vi "classeParCarton.vi"(11 "Tableau":string[][](array[string])=[["484147311015190508  ", "06.05.2015 09:48:00", "1866", "155915", "1", "1", "1", "11", "0"], ["484147311015190518  ", "06.05.2015 09:50:00", "1866", "155915", "1", "1", "1", "12", "0"], ["484147311015190505  ", "06.05.2015 09:38:00", "1866", "155915", "1", "1", "1", "5", "0"], ["484147311015190517  ", "06.05.2015 09:52:00", "1866", "155915", "1", "1", "1", "13", "0"], ["484147311015190506  ", "06.05.2015 09:50:00", "1866", "155915", "1", "1", "1", "12", "0"], ["484147311015190522  ", "06.05.2015 09:50:00", "1866", "155915", "1", "1", "1", "12", "0"], ["484147311015190533  ", "06.05.2015 09:41:00", "1866", "155915", "1", "1", "1", "7", "0"], ["484147311015190507  ", "06.05.2015 09:43:00", "1866", "155915", "1", "1", "1", "8", "0"], ["484147311015190550  ", "06.05.2015 09:50:00", "1866", "155915", "1", "1", "1", "12", "0"], ["484147311015190534  ", "06.05.2015 09:52:00", "1866", "155915", "1", "1", "1", "13", "0"], ["484147311015190535  ", "06.05.2015 09:40:00", "1866", "155915", "1", "1", "1", "6", "0"], ["484147311015190536  ", "06.05.2015 09:50:00", "1866", "155915", "1", "1", "1", "12", "0"], ["484147311015190537  ", "06.05.2015 09:53:00", "1866", "155915", "1", "1", "1", "13", "0"], ["484147311015190538  ", "06.05.2015 09:50:00", "1866", "155915", "1", "1", "1", "12", "0"], ["484147311015190551  ", "06.05.2015 09:53:00", "1866", "155915", "1", "1", "1", "13", "0"], ["484147311015190552  ", "06.05.2015 09:52:00", "1866", "155915", "1", "1", "1", "13", "0"], ["484147311015190539  ", "06.05.2015 09:53:00", "1866", "155915", "1", "1", "1", "13", "0"], ["484147311015190549  ", "06.05.2015 09:50:00", "1866", "155915", "1", "1", "1", "12", "0"], ["484147311015190540  ", "06.05.2015 09:38:00", "1866", "155915", "1", "1", "1", "5", "0"], ["484147311015190541  ", "06.05.2015 09:52:00", "1866", "155915", "1", "1", "1", "13", "0"], ["484147311015190527  ", "06.05.2015 09:50:00", "1866", "155915", "1", "1", "1", "12", "0"], ["484147311015190531  ", "06.05.2015 09:51:00", "1866", "155915", "1", "1", "1", "13", "0"], ["484147311015190525  ", "06.05.2015 09:41:00", "1866", "155915", "1", "1", "1", "7", "0"], ["484147311015190545  ", "06.05.2015 09:50:00", "1866", "155915", "1", "1", "1", "12", "0"], ["484147311015190546  ", "06.05.2015 09:53:00", "1866", "155915", "1", "1", "1", "13", "0"], ["484147311015190547  ", "06.05.2015 09:49:00", "1866", "155915", "1", "1", "1", "11", "0"], ["484147311015190521  ", "06.05.2015 09:48:00", "1866", "155915", "1", "1", "1", "11", "0"], ["484147311015190574  ", "06.05.2015 09:35:00", "1866", "155915", "1", "1", "1", "3", "0"], ["484147311015190548  ", "06.05.2015 09:38:00", "1866", "155915", "1", "1", "1", "5", "0"], ["484147311015190520  ", "06.05.2015 09:34:00", "1866", "155915", "1", "1", "1", "2", "0"], ["484147311015190577  ", "06.05.2015 09:32:00", "1866", "155915", "1", "1", "1", "1", "0"], ["484147311015190573  ", "06.05.2015 09:37:00", "1866", "155915", "1", "1", "1", "4", "0"], ["484147311015190572  ", "06.05.2015 09:31:00", "1866", "155915", "1", "1", "1", "1", "0"], ["484147311015190569  ", "06.05.2015 09:39:00", "1866", "155915", "1", "1", "1", "6", "0"], ["484147311015190501  ", "06.05.2015 09:40:00", "1866", "155915", "1", "1", "1", "6", "0"], ["484147311015190503  ", "06.05.2015 09:39:00", "1866", "155915", "1", "1", "1", "6", "0"], ["484147311015190584  ", "06.05.2015 09:38:00", "1866", "155915", "1", "1", "1", "5", "0"], ["484147311015190583  ", "06.05.2015 09:32:00", "1866", "155915", "1", "1", "1", "1", "0"], ["484147311015190568  ", "06.05.2015 09:50:00", "1866", "155915", "1", "1", "1", "12", "0"], ["484147311015190567  ", "06.05.2015 09:40:00", "1866", "155915", "1", "1", "1", "6", "0"], ["484147311015190519  ", "06.05.2015 09:34:00", "1866", "155915", "1", "1", "1", "2", "0"], ["484147311015190566  ", "06.05.2015 09:48:00", "1866", "155915", "1", "1", "1", "11", "0"], ["484147311015190565  ", "06.05.2015 09:34:00", "1866", "155915", "1", "1", "1", "2", "0"], ["484147311015190581  ", "06.05.2015 09:46:00", "1866", "155915", "1", "1", "1", "10", "0"], ["484147311015190564  ", "06.05.2015 09:32:00", "1866", "155915", "1", "1", "1", "1", "0"], ["484147311015190575  ", "06.05.2015 09:42:00", "1866", "155915", "1", "1", "1", "7", "0"], ["484147311015190576  ", "06.05.2015 09:34:00", "1866", "155915", "1", "1", "1", "2", "0"], ["484147311015190578  ", "06.05.2015 09:34:00", "1866", "155915", "1", "1", "1", "2", "0"], ["484147311015190563  ", "06.05.2015 09:43:00", "1866", "155915", "1", "1", "1", "8", "0"], ["484147311015190561  ", "06.05.2015 09:45:00", "1866", "155915", "1", "1", "1", "9", "0"], ["484147311015190579  ", "06.05.2015 09:32:00", "1866", "155915", "1", "1", "1", "1", "0"], ["484147311015190562  ", "06.05.2015 09:32:00", "1866", "155915", "1", "1", "1", "1", "0"], ["484147311015190582  ", "06.05.2015 09:42:00", "1866", "155915", "1", "1", "1", "8", "0"], ["484147311015190560  ", "06.05.2015 09:32:00", "1866", "155915", "1", "1", "1", "1", "0"], ["484147311015190587  ", "06.05.2015 09:34:00", "1866", "155915", "1", "1", "1", "2", "0"], ["484147311015190590  ", "06.05.2015 09:34:00", "1866", "155915", "1", "1", "1", "2", "0"], ["484147311015190589  ", "06.05.2015 09:43:00", "1866", "155915", "1", "1", "1", "8", "0"], ["484147311015190559  ", "06.05.2015 09:33:00", "1866", "155915", "1", "1", "1", "1", "0"], ["484147311015190585  ", "06.05.2015 09:33:00", "1866", "155915", "1", "1", "1", "2", "0"], ["484147311015190558  ", "06.05.2015 09:42:00", "1866", "155915", "1", "1", "1", "7", "0"], ["484147311015190586  ", "06.05.2015 09:43:00", "1866", "155915", "1", "1", "1", "8", "0"], ["484147311015190588  ", "06.05.2015 09:45:00", "1866", "155915", "1", "1", "1", "9", "0"], ["484147311015190603  ", "06.05.2015 09:38:00", "1866", "155915", "1", "1", "1", "5", "0"], ["484147311015190594  ", "06.05.2015 09:33:00", "1866", "155915", "1", "1", "1", "2", "0"], ["484147311015190593  ", "06.05.2015 09:33:00", "1866", "155915", "1", "1", "1", "2", "0"], ["484147311015190604  ", "06.05.2015 09:39:00", "1866", "155915", "1", "1", "1", "6", "0"], ["484147311015190595  ", "06.05.2015 09:34:00", "1866", "155915", "1", "1", "1", "2", "0"], ["484147311015190596  ", "06.05.2015 09:32:00", "1866", "155915", "1", "1", "1", "1", "0"], ["484147311015190597  ", "06.05.2015 09:32:00", "1866", "155915", "1", "1", "1", "1", "0"], ["484147311015190606  ", "06.05.2015 09:31:00", "1866", "155915", "1", "1", "1", "1", "0"], ["484147311015190598  ", "06.05.2015 09:32:00", "1866", "155915", "1", "1", "1", "1", "0"], ["484147311015190605  ", "06.05.2015 09:35:00", "1866", "155915", "1", "1", "1", "3", "0"], ["484147311015190599  ", "06.05.2015 09:32:00", "1866", "155915", "1", "1", "1", "1", "0"], ["484147311015190608  ", "06.05.2015 09:34:00", "1866", "155915", "1", "1", "1", "2", "0"], ["484147311015190600  ", "06.05.2015 09:32:00", "1866", "155915", "1", "1", "1", "1", "0"], ["484147311015190556  ", "06.05.2015 09:31:00", "1866", "155915", "1", "1", "1", "1", "0"], ["484147311015190555  ", "06.05.2015 09:32:00", "1866", "155915", "1", "1", "1", "1", "0"], ["484147311015190602  ", "06.05.2015 09:34:00", "1866", "155915", "1", "1", "1", "2", "0"], ["484147311015190609  ", "06.05.2015 09:33:00", "1866", "155915", "1", "1", "1", "2", "0"], ["484147311015190610  ", "06.05.2015 09:32:00", "1866", "155915", "1", "1", "1", "1", "0"], ["484147311015190611  ", "06.05.2015 09:33:00", "1866", "155915", "1", "1", "1", "2", "0"], ["484147311015190554  ", "06.05.2015 09:38:00", "1866", "155915", "1", "1", "1", "5", "0"], ["484147311015190613  ", "06.05.2015 09:40:00", "1866", "155915", "1", "1", "1", "6", "0"], ["484147311015190612  ", "06.05.2015 09:55:00", "1866", "155915", "1", "1", "1", "14", "0"], ["484147311015190623  ", "06.05.2015 09:32:00", "1866", "155915", "1", "1", "1", "1", "0"], ["484147311015190614  ", "06.05.2015 09:41:00", "1866", "155915", "1", "1", "1", "7", "0"], ["484147311015190625  ", "06.05.2015 09:32:00", "1866", "155915", "1", "1", "1", "1", "0"], ["484147311015190615  ", "06.05.2015 09:35:00", "1866", "155915", "1", "1", "1", "3", "0"], ["484147311015190617  ", "06.05.2015 09:37:00", "1866", "155915", "1", "1", "1", "4", "0"], ["484147311015190616  ", "06.05.2015 09:41:00", "1866", "155915", "1", "1", "1", "7", "0"], ["484147311015190618  ", "06.05.2015 09:37:00", "1866", "155915", "1", "1", "1", "4", "0"], ["484147311015190619  ", "06.05.2015 09:39:00", "1866", "155915", "1", "1", "1", "6", "0"], ["484147311015190627  ", "06.05.2015 09:40:00", "1866", "155915", "1", "1", "1", "6", "0"], ["484147311015190620  ", "06.05.2015 09:46:00", "1866", "155915", "1", "1", "1", "10", "0"], ["484147311015190629  ", "06.05.2015 09:46:00", "1866", "155915", "1", "1", "1", "10", "0"], ["484147311015190633  ", "06.05.2015 09:38:00", "1866", "155915", "1", "1", "1", "5", "0"], ["484147311015190601  ", "06.05.2015 09:46:00", "1866", "155915", "1", "1", "1", "10", "0"], ["484147311015190635  ", "06.05.2015 09:39:00", "1866", "155915", "1", "1", "1", "6", "0"], ["484147311015190637  ", "06.05.2015 09:45:00", "1866", "155915", "1", "1", "1", "9", "0"], ["484147311015190636  ", "06.05.2015 09:49:00", "1866", "155915", "1", "1", "1", "11", "0"], ["484147311015190667  ", "06.05.2015 09:39:00", "1866", "155915", "1", "1", "1", "6", "0"], ["484147311015180237  ", "06.05.2015 10:00:00", "1866", "155915", "1", "1", "1", "16", "0"], ["484147311015180267  ", "06.05.2015 09:58:00", "1866", "155915", "1", "1", "1", "15", "0"], ["484147311015180419  ", "06.05.2015 10:01:00", "1866", "155915", "1", "1", "1", "16", "0"], ["484147311015180644  ", "06.05.2015 09:50:00", "1866", "155915", "1", "1", "1", "12", "0"], ["484147311015180688  ", "06.05.2015 10:01:00", "1866", "155915", "1", "1", "1", "16", "0"], ["484147311015180709  ", "06.05.2015 10:01:00", "1866", "155915", "1", "1", "1", "16", "0"], ["484147311015180701  ", "06.05.2015 09:55:00", "1866", "155915", "1", "1", "1", "14", "0"], ["484147311015180703  ", "06.05.2015 10:01:00", "1866", "155915", "1", "1", "1", "16", "0"], ["484147311015180707  ", "06.05.2015 09:56:00", "1866", "155915", "1", "1", "1", "14", "0"], ["484147311015180718  ", "06.05.2015 10:00:00", "1866", "155915", "1", "1", "1", "16", "0"], ["484147311015180717  ", "06.05.2015 09:57:00", "1866", "155915", "1", "1", "1", "15", "0"], ["484147311015180715  ", "06.05.2015 09:55:00", "1866", "155915", "1", "1", "1", "14", "0"], ["484147311015180726  ", "06.05.2015 09:56:00", "1866", "155915", "1", "1", "1", "14", "0"], ["484147311015180728  ", "06.05.2015 09:56:00", "1866", "155915", "1", "1", "1", "14", "0"], ["484147311015180737  ", "06.05.2015 10:00:00", "1866", "155915", "1", "1", "1", "16", "0"], ["484147311015190019  ", "06.05.2015 09:33:00", "1866", "155915", "1", "1", "1", "2", "0"], ["484147311015190016  ", "06.05.2015 09:47:00", "1866", "155915", "1", "1", "1", "10", "0"], ["484147311015190022  ", "06.05.2015 09:43:00", "1866", "155915", "1", "1", "1", "8", "0"], ["484147311015190027  ", "06.05.2015 09:48:00", "1866", "155915", "1", "1", "1", "11", "0"], ["484147311015190035  ", "06.05.2015 10:00:00", "1866", "155915", "1", "1", "1", "16", "0"], ["484147311015190044  ", "06.05.2015 10:01:00", "1866", "155915", "1", "1", "1", "16", "0"], ["484147311015190046  ", "06.05.2015 09:58:00", "1866", "155915", "1", "1", "1", "15", "0"], ["484147311015190045  ", "06.05.2015 09:57:00", "1866", "155915", "1", "1", "1", "15", "0"], ["484147311015190057  ", "06.05.2015 09:58:00", "1866", "155915", "1", "1", "1", "15", "0"], ["484147311015190055  ", "06.05.2015 09:33:00", "1866", "155915", "1", "1", "1", "2", "0"], ["484147311015190056  ", "06.05.2015 09:58:00", "1866", "155915", "1", "1", "1", "15", "0"], ["484147311015190052  ", "06.05.2015 09:56:00", "1866", "155915", "1", "1", "1", "14", "0"], ["484147311015190059  ", "06.05.2015 09:58:00", "1866", "155915", "1", "1", "1", "15", "0"], ["484147311015190060  ", "06.05.2015 09:59:00", "1866", "155915", "1", "1", "1", "15", "0"], ["484147311015190064  ", "06.05.2015 09:58:00", "1866", "155915", "1", "1", "1", "15", "0"], ["484147311015190068  ", "06.05.2015 09:47:00", "1866", "155915", "1", "1", "1", "10", "0"], ["484147311015190084  ", "06.05.2015 09:59:00", "1866", "155915", "1", "1", "1", "15", "0"], ["484147311015190081  ", "06.05.2015 09:59:00", "1866", "155915", "1", "1", "1", "15", "0"], ["484147311015190082  ", "06.05.2015 10:00:00", "1866", "155915", "1", "1", "1", "16", "0"], ["484147311015190098  ", "06.05.2015 09:56:00", "1866", "155915", "1", "1", "1", "14", "0"], ["484147311015190096  ", "06.05.2015 09:59:00", "1866", "155915", "1", "1", "1", "15", "0"], ["484147311015190091  ", "06.05.2015 09:56:00", "1866", "155915", "1", "1", "1", "14", "0"], ["484147311015190118  ", "06.05.2015 09:55:00", "1866", "155915", "1", "1", "1", "14", "0"], ["484147311015190117  ", "06.05.2015 09:40:00", "1866", "155915", "1", "1", "1", "6", "0"], ["484147311015190113  ", "06.05.2015 10:00:00", "1866", "155915", "1", "1", "1", "16", "0"], ["484147311015190111  ", "06.05.2015 10:01:00", "1866", "155915", "1", "1", "1", "16", "0"], ["484147311015190108  ", "06.05.2015 10:00:00", "1866", "155915", "1", "1", "1", "16", "0"], ["484147311015190135  ", "06.05.2015 09:59:00", "1866", "155915", "1", "1", "1", "15", "0"], ["484147311015190133  ", "06.05.2015 10:00:00", "1866", "155915", "1", "1", "1", "16", "0"], ["484147311015190131  ", "06.05.2015 09:41:00", "1866", "155915", "1", "1", "1", "7", "0"], ["484147311015190129  ", "06.05.2015 09:56:00", "1866", "155915", "1", "1", "1", "14", "0"], ["484147311015190123  ", "06.05.2015 09:57:00", "1866", "155915", "1", "1", "1", "15", "0"], ["484147311015190121  ", "06.05.2015 09:57:00", "1866", "155915", "1", "1", "1", "15", "0"], ["484147311015190124  ", "06.05.2015 09:58:00", "1866", "155915", "1", "1", "1", "15", "0"], ["484147311015190126  ", "06.05.2015 10:01:00", "1866", "155915", "1", "1", "1", "16", "0"], ["484147311015190132  ", "06.05.2015 10:00:00", "1866", "155915", "1", "1", "1", "16", "0"], ["484147311015190150  ", "06.05.2015 09:59:00", "1866", "155915", "1", "1", "1", "15", "0"], ["484147311015190146  ", "06.05.2015 09:58:00", "1866", "155915", "1", "1", "1", "15", "0"], ["484147311015190149  ", "06.05.2015 09:57:00", "1866", "155915", "1", "1", "1", "15", "0"], ["484147311015190145  ", "06.05.2015 09:48:00", "1866", "155915", "1", "1", "1", "11", "0"], ["484147311015190159  ", "06.05.2015 09:57:00", "1866", "155915", "1", "1", "1", "15", "0"], ["484147311015190183  ", "06.05.2015 09:56:00", "1866", "155915", "1", "1", "1", "14", "0"], ["484147311015190181  ", "06.05.2015 09:56:00", "1866", "155915", "1", "1", "1", "14", "0"], ["484147311015190180  ", "06.05.2015 09:55:00", "1866", "155915", "1", "1", "1", "14", "0"], ["484147311015190179  ", "06.05.2015 10:01:00", "1866", "155915", "1", "1", "1", "16", "0"], ["484147311015190177  ", "06.05.2015 09:48:00", "1866", "155915", "1", "1", "1", "11", "0"], ["484147311015190168  ", "06.05.2015 09:58:00", "1866", "155915", "1", "1", "1", "15", "0"], ["484147311015190173  ", "06.05.2015 09:56:00", "1866", "155915", "1", "1", "1", "14", "0"], ["484147311015190175  ", "06.05.2015 09:58:00", "1866", "155915", "1", "1", "1", "15", "0"], ["484147311015190193  ", "06.05.2015 10:01:00", "1866", "155915", "1", "1", "1", "16", "0"], ["484147311015190194  ", "06.05.2015 09:58:00", "1866", "155915", "1", "1", "1", "15", "0"], ["484147311015190197  ", "06.05.2015 10:01:00", "1866", "155915", "1", "1", "1", "16", "0"], ["484147311015190196  ", "06.05.2015 09:59:00", "1866", "155915", "1", "1", "1", "15", "0"], ["484147311015190198  ", "06.05.2015 09:56:00", "1866", "155915", "1", "1", "1", "14", "0"], ["484147311015190188  ", "06.05.2015 09:59:00", "1866", "155915", "1", "1", "1", "15", "0"], ["484147311015190218  ", "06.05.2015 09:39:00", "1866", "155915", "1", "1", "1", "5", "0"], ["484147311015190215  ", "06.05.2015 10:01:00", "1866", "155915", "1", "1", "1", "16", "0"], ["484147311015190290  ", "06.05.2015 09:42:00", "1866", "155915", "1", "1", "1", "7", "0"], ["484147311015190288  ", "06.05.2015 09:50:00", "1866", "155915", "1", "1", "1", "12", "0"], ["484147311015190297  ", "06.05.2015 09:46:00", "1866", "155915", "1", "1", "1", "10", "0"], ["484147311015190314  ", "06.05.2015 09:45:00", "1866", "155915", "1", "1", "1", "9", "0"], ["484147311015190313  ", "06.05.2015 09:42:00", "1866", "155915", "1", "1", "1", "8", "0"], ["484147311015190312  ", "06.05.2015 09:41:00", "1866", "155915", "1", "1", "1", "7", "0"], ["484147311015190311  ", "06.05.2015 09:45:00", "1866", "155915", "1", "1", "1", "9", "0"], ["484147311015190310  ", "06.05.2015 09:42:00", "1866", "155915", "1", "1", "1", "7", "0"], ["484147311015190303  ", "06.05.2015 09:42:00", "1866", "155915", "1", "1", "1", "7", "0"], ["484147311015190306  ", "06.05.2015 09:42:00", "1866", "155915", "1", "1", "1", "8", "0"], ["484147311015190305  ", "06.05.2015 09:45:00", "1866", "155915", "1", "1", "1", "9", "0"], ["484147311015190304  ", "06.05.2015 09:45:00", "1866", "155915", "1", "1", "1", "9", "0"], ["484147311015190307  ", "06.05.2015 09:42:00", "1866", "155915", "1", "1", "1", "8", "0"], ["484147311015190308  ", "06.05.2015 09:41:00", "1866", "155915", "1", "1", "1", "7", "0"], ["484147311015190309  ", "06.05.2015 09:45:00", "1866", "155915", "1", "1", "1", "9", "0"], ["484147311015190326  ", "06.05.2015 09:42:00", "1866", "155915", "1", "1", "1", "7", "0"], ["484147311015190328  ", "06.05.2015 09:34:00", "1866", "155915", "1", "1", "1", "2", "0"], ["484147311015190329  ", "06.05.2015 09:40:00", "1866", "155915", "1", "1", "1", "6", "0"], ["484147311015190330  ", "06.05.2015 09:46:00", "1866", "155915", "1", "1", "1", "10", "0"], ["484147311015190331  ", "06.05.2015 09:45:00", "1866", "155915", "1", "1", "1", "9", "0"], ["484147311015190317  ", "06.05.2015 09:43:00", "1866", "155915", "1", "1", "1", "8", "0"], ["484147311015190316  ", "06.05.2015 09:45:00", "1866", "155915", "1", "1", "1", "9", "0"], ["484147311015190318  ", "06.05.2015 09:49:00", "1866", "155915", "1", "1", "1", "12", "0"], ["484147311015190320  ", "06.05.2015 09:34:00", "1866", "155915", "1", "1", "1", "2", "0"], ["484147311015190321  ", "06.05.2015 09:46:00", "1866", "155915", "1", "1", "1", "10", "0"], ["484147311015190322  ", "06.05.2015 09:45:00", "1866", "155915", "1", "1", "1", "9", "0"], ["484147311015190323  ", "06.05.2015 09:45:00", "1866", "155915", "1", "1", "1", "9", "0"], ["484147311015190347  ", "06.05.2015 09:43:00", "1866", "155915", "1", "1", "1", "8", "0"], ["484147311015190346  ", "06.05.2015 09:46:00", "1866", "155915", "1", "1", "1", "10", "0"], ["484147311015190345  ", "06.05.2015 09:36:00", "1866", "155915", "1", "1", "1", "3", "0"], ["484147311015190344  ", "06.05.2015 09:45:00", "1866", "155915", "1", "1", "1", "9", "0"], ["484147311015190343  ", "06.05.2015 09:44:00", "1866", "155915", "1", "1", "1", "9", "0"], ["484147311015190341  ", "06.05.2015 09:44:00", "1866", "155915", "1", "1", "1", "9", "0"], ["484147311015190340  ", "06.05.2015 09:46:00", "1866", "155915", "1", "1", "1", "10", "0"], ["484147311015190332  ", "06.05.2015 09:45:00", "1866", "155915", "1", "1", "1", "9", "0"], ["484147311015190333  ", "06.05.2015 09:35:00", "1866", "155915", "1", "1", "1", "3", "0"], ["484147311015190334  ", "06.05.2015 09:45:00", "1866", "155915", "1", "1", "1", "9", "0"], ["484147311015190335  ", "06.05.2015 09:46:00", "1866", "155915", "1", "1", "1", "10", "0"], ["484147311015190336  ", "06.05.2015 09:45:00", "1866", "155915", "1", "1", "1", "9", "0"], ["484147311015190337  ", "06.05.2015 09:33:00", "1866", "155915", "1", "1", "1", "2", "0"], ["484147311015190339  ", "06.05.2015 09:42:00", "1866", "155915", "1", "1", "1", "7", "0"], ["484147311015190348  ", "06.05.2015 09:43:00", "1866", "155915", "1", "1", "1", "8", "0"], ["484147311015190349  ", "06.05.2015 09:46:00", "1866", "155915", "1", "1", "1", "10", "0"], ["484147311015190350  ", "06.05.2015 09:43:00", "1866", "155915", "1", "1", "1", "8", "0"], ["484147311015190351  ", "06.05.2015 09:45:00", "1866", "155915", "1", "1", "1", "9", "0"], ["484147311015190352  ", "06.05.2015 09:45:00", "1866", "155915", "1", "1", "1", "9", "0"], ["484147311015190353  ", "06.05.2015 09:33:00", "1866", "155915", "1", "1", "1", "2", "0"], ["484147311015190354  ", "06.05.2015 09:35:00", "1866", "155915", "1", "1", "1", "3", "0"], ["484147311015190360  ", "06.05.2015 09:37:00", "1866", "155915", "1", "1", "1", "4", "0"], ["484147311015190355  ", "06.05.2015 09:32:00", "1866", "155915", "1", "1", "1", "1", "0"], ["484147311015190361  ", "06.05.2015 09:37:00", "1866", "155915", "1", "1", "1", "4", "0"], ["484147311015190356  ", "06.05.2015 09:41:00", "1866", "155915", "1", "1", "1", "7", "0"], ["484147311015190362  ", "06.05.2015 09:39:00", "1866", "155915", "1", "1", "1", "5", "0"], ["484147311015190357  ", "06.05.2015 09:37:00", "1866", "155915", "1", "1", "1", "4", "0"], ["484147311015190363  ", "06.05.2015 09:36:00", "1866", "155915", "1", "1", "1", "4", "0"], ["484147311015190358  ", "06.05.2015 09:44:00", "1866", "155915", "1", "1", "1", "9", "0"], ["484147311015190372  ", "06.05.2015 09:35:00", "1866", "155915", "1", "1", "1", "3", "0"], ["484147311015190371  ", "06.05.2015 09:36:00", "1866", "155915", "1", "1", "1", "4", "0"], ["484147311015190373  ", "06.05.2015 09:36:00", "1866", "155915", "1", "1", "1", "3", "0"], ["484147311015190370  ", "06.05.2015 09:41:00", "1866", "155915", "1", "1", "1", "7", "0"], ["484147311015190381  ", "06.05.2015 09:37:00", "1866", "155915", "1", "1", "1", "4", "0"], ["484147311015190380  ", "06.05.2015 09:36:00", "1866", "155915", "1", "1", "1", "3", "0"], ["484147311015190386  ", "06.05.2015 09:35:00", "1866", "155915", "1", "1", "1", "3", "0"], ["484147311015190382  ", "06.05.2015 09:45:00", "1866", "155915", "1", "1", "1", "9", "0"], ["484147311015190387  ", "06.05.2015 09:35:00", "1866", "155915", "1", "1", "1", "3", "0"], ["484147311015190369  ", "06.05.2015 09:41:00", "1866", "155915", "1", "1", "1", "7", "0"], ["484147311015190375  ", "06.05.2015 09:48:00", "1866", "155915", "1", "1", "1", "11", "0"], ["484147311015190376  ", "06.05.2015 09:36:00", "1866", "155915", "1", "1", "1", "3", "0"], ["484147311015190367  ", "06.05.2015 09:40:00", "1866", "155915", "1", "1", "1", "6", "0"], ["484147311015190377  ", "06.05.2015 09:40:00", "1866", "155915", "1", "1", "1", "6", "0"], ["484147311015190399  ", "06.05.2015 09:48:00", "1866", "155915", "1", "1", "1", "11", "0"], ["484147311015190395  ", "06.05.2015 09:49:00", "1866", "155915", "1", "1", "1", "12", "0"], ["484147311015190397  ", "06.05.2015 09:35:00", "1866", "155915", "1", "1", "1", "3", "0"], ["484147311015190378  ", "06.05.2015 09:39:00", "1866", "155915", "1", "1", "1", "6", "0"], ["484147311015190364  ", "06.05.2015 09:39:00", "1866", "155915", "1", "1", "1", "5", "0"], ["484147311015190393  ", "06.05.2015 09:40:00", "1866", "155915", "1", "1", "1", "6", "0"], ["484147311015190379  ", "06.05.2015 09:40:00", "1866", "155915", "1", "1", "1", "6", "0"], ["484147311015190389  ", "06.05.2015 09:40:00", "1866", "155915", "1", "1", "1", "6", "0"], ["484147311015190365  ", "06.05.2015 09:39:00", "1866", "155915", "1", "1", "1", "5", "0"], ["484147311015190412  ", "06.05.2015 09:38:00", "1866", "155915", "1", "1", "1", "5", "0"], ["484147311015190411  ", "06.05.2015 09:40:00", "1866", "155915", "1", "1", "1", "6", "0"], ["484147311015190409  ", "06.05.2015 09:38:00", "1866", "155915", "1", "1", "1", "5", "0"], ["484147311015190408  ", "06.05.2015 09:41:00", "1866", "155915", "1", "1", "1", "7", "0"], ["484147311015190407  ", "06.05.2015 09:55:00", "1866", "155915", "1", "1", "1", "14", "0"], ["484147311015190391  ", "06.05.2015 09:53:00", "1866", "155915", "1", "1", "1", "13", "0"], ["484147311015190400  ", "06.05.2015 09:35:00", "1866", "155915", "1", "1", "1", "3", "0"], ["484147311015190406  ", "06.05.2015 09:48:00", "1866", "155915", "1", "1", "1", "11", "0"], ["484147311015190426  ", "06.05.2015 09:49:00", "1866", "155915", "1", "1", "1", "12", "0"], ["484147311015190425  ", "06.05.2015 09:38:00", "1866", "155915", "1", "1", "1", "5", "0"], ["484147311015190427  ", "06.05.2015 09:42:00", "1866", "155915", "1", "1", "1", "7", "0"], ["484147311015190405  ", "06.05.2015 09:47:00", "1866", "155915", "1", "1", "1", "10", "0"], ["484147311015190430  ", "06.05.2015 09:35:00", "1866", "155915", "1", "1", "1", "3", "0"], ["484147311015190429  ", "06.05.2015 09:53:00", "1866", "155915", "1", "1", "1", "13", "0"], ["484147311015190410  ", "06.05.2015 09:47:00", "1866", "155915", "1", "1", "1", "10", "0"], ["484147311015190401  ", "06.05.2015 09:48:00", "1866", "155915", "1", "1", "1", "11", "0"], ["484147311015190404  ", "06.05.2015 09:37:00", "1866", "155915", "1", "1", "1", "4", "0"], ["484147311015190396  ", "06.05.2015 09:55:00", "1866", "155915", "1", "1", "1", "14", "0"], ["484147311015190394  ", "06.05.2015 09:38:00", "1866", "155915", "1", "1", "1", "5", "0"], ["484147311015190402  ", "06.05.2015 09:38:00", "1866", "155915", "1", "1", "1", "5", "0"], ["484147311015190390  ", "06.05.2015 09:37:00", "1866", "155915", "1", "1", "1", "4", "0"], ["484147311015190388  ", "06.05.2015 09:39:00", "1866", "155915", "1", "1", "1", "5", "0"], ["484147311015190436  ", "06.05.2015 09:42:00", "1866", "155915", "1", "1", "1", "8", "0"], ["484147311015190433  ", "06.05.2015 09:55:00", "1866", "155915", "1", "1", "1", "14", "0"], ["484147311015190434  ", "06.05.2015 09:41:00", "1866", "155915", "1", "1", "1", "7", "0"], ["484147311015190438  ", "06.05.2015 09:53:00", "1866", "155915", "1", "1", "1", "13", "0"], ["484147311015190392  ", "06.05.2015 09:55:00", "1866", "155915", "1", "1", "1", "14", "0"], ["484147311015190432  ", "06.05.2015 09:41:00", "1866", "155915", "1", "1", "1", "7", "0"], ["484147311015190431  ", "06.05.2015 09:55:00", "1866", "155915", "1", "1", "1", "14", "0"], ["484147311015190435  ", "06.05.2015 09:38:00", "1866", "155915", "1", "1", "1", "5", "0"], ["484147311015190422  ", "06.05.2015 09:54:00", "1866", "155915", "1", "1", "1", "14", "0"], ["484147311015190423  ", "06.05.2015 09:55:00", "1866", "155915", "1", "1", "1", "14", "0"], ["484147311015190421  ", "06.05.2015 09:41:00", "1866", "155915", "1", "1", "1", "7", "0"], ["484147311015190420  ", "06.05.2015 09:37:00", "1866", "155915", "1", "1", "1", "4", "0"], ["484147311015190424  ", "06.05.2015 09:52:00", "1866", "155915", "1", "1", "1", "13", "0"], ["484147311015190418  ", "06.05.2015 09:52:00", "1866", "155915", "1", "1", "1", "13", "0"], ["484147311015190419  ", "06.05.2015 09:38:00", "1866", "155915", "1", "1", "1", "5", "0"], ["484147311015190417  ", "06.05.2015 09:46:00", "1866", "155915", "1", "1", "1", "10", "0"], ["484147311015190439  ", "06.05.2015 09:53:00", "1866", "155915", "1", "1", "1", "13", "0"], ["484147311015190416  ", "06.05.2015 09:35:00", "1866", "155915", "1", "1", "1", "3", "0"], ["484147311015190414  ", "06.05.2015 09:49:00", "1866", "155915", "1", "1", "1", "11", "0"], ["484147311015190441  ", "06.05.2015 09:40:00", "1866", "155915", "1", "1", "1", "6", "0"], ["484147311015190415  ", "06.05.2015 09:52:00", "1866", "155915", "1", "1", "1", "13", "0"], ["484147311015190442  ", "06.05.2015 09:52:00", "1866", "155915", "1", "1", "1", "13", "0"], ["484147311015190440  ", "06.05.2015 09:36:00", "1866", "155915", "1", "1", "1", "4", "0"], ["484147311015190443  ", "06.05.2015 09:54:00", "1866", "155915", "1", "1", "1", "14", "0"], ["484147311015190413  ", "06.05.2015 09:37:00", "1866", "155915", "1", "1", "1", "4", "0"], ["484147311015190446  ", "06.05.2015 09:37:00", "1866", "155915", "1", "1", "1", "4", "0"], ["484147311015190444  ", "06.05.2015 09:53:00", "1866", "155915", "1", "1", "1", "13", "0"], ["484147311015190466  ", "06.05.2015 09:43:00", "1866", "155915", "1", "1", "1", "8", "0"], ["484147311015190437  ", "06.05.2015 09:40:00", "1866", "155915", "1", "1", "1", "6", "0"], ["484147311015190463  ", "06.05.2015 09:42:00", "1866", "155915", "1", "1", "1", "7", "0"], ["484147311015190459  ", "06.05.2015 09:48:00", "1866", "155915", "1", "1", "1", "11", "0"], ["484147311015190462  ", "06.05.2015 09:53:00", "1866", "155915", "1", "1", "1", "13", "0"], ["484147311015190655  ", "06.05.2015 09:48:00", "1866", "155915", "1", "1", "1", "11", "0"], ["484147311015190634  ", "06.05.2015 09:43:00", "1866", "155915", "1", "1", "1", "8", "0"], ["484147311015190657  ", "06.05.2015 09:39:00", "1866", "155915", "1", "1", "1", "6", "0"], ["484147311015190630  ", "06.05.2015 09:40:00", "1866", "155915", "1", "1", "1", "6", "0"], ["484147311015190632  ", "06.05.2015 09:47:00", "1866", "155915", "1", "1", "1", "10", "0"], ["484147311015190659  ", "06.05.2015 09:44:00", "1866", "155915", "1", "1", "1", "9", "0"], ["484147311015190661  ", "06.05.2015 09:46:00", "1866", "155915", "1", "1", "1", "10", "0"], ["484147311015190628  ", "06.05.2015 09:43:00", "1866", "155915", "1", "1", "1", "8", "0"], ["484147311015190663  ", "06.05.2015 09:44:00", "1866", "155915", "1", "1", "1", "9", "0"], ["484147311015190650  ", "06.05.2015 09:50:00", "1866", "155915", "1", "1", "1", "12", "0"], ["484147311015190652  ", "06.05.2015 09:48:00", "1866", "155915", "1", "1", "1", "11", "0"], ["484147311015190665  ", "06.05.2015 09:47:00", "1866", "155915", "1", "1", "1", "10", "0"], ["484147311015190649  ", "06.05.2015 09:32:00", "1866", "155915", "1", "1", "1", "1", "0"], ["484147311015190648  ", "06.05.2015 09:48:00", "1866", "155915", "1", "1", "1", "11", "0"], ["484147311015190647  ", "06.05.2015 09:48:00", "1866", "155915", "1", "1", "1", "11", "0"], ["484147311015190622  ", "06.05.2015 09:47:00", "1866", "155915", "1", "1", "1", "10", "0"], ["484147311015190644  ", "06.05.2015 09:31:00", "1866", "155915", "1", "1", "1", "1", "0"], ["484147311015190645  ", "06.05.2015 09:50:00", "1866", "155915", "1", "1", "1", "12", "0"], ["484147311015190654  ", "06.05.2015 09:42:00", "1866", "155915", "1", "1", "1", "8", "0"], ["484147311015190624  ", "06.05.2015 09:43:00", "1866", "155915", "1", "1", "1", "8", "0"], ["484147311015190642  ", "06.05.2015 09:42:00", "1866", "155915", "1", "1", "1", "7", "0"], ["484147311015190656  ", "06.05.2015 09:31:00", "1866", "155915", "1", "1", "1", "1", "0"], ["484147311015190641  ", "06.05.2015 09:41:00", "1866", "155915", "1", "1", "1", "7", "0"], ["484147311015190658  ", "06.05.2015 09:33:00", "1866", "155915", "1", "1", "1", "2", "0"], ["484147311015190640  ", "06.05.2015 09:43:00", "1866", "155915", "1", "1", "1", "8", "0"], ["484147311015190662  ", "06.05.2015 09:43:00", "1866", "155915", "1", "1", "1", "8", "0"], ["484147311015190660  ", "06.05.2015 09:32:00", "1866", "155915", "1", "1", "1", "1", "0"], ["484147311015190664  ", "06.05.2015 09:33:00", "1866", "155915", "1", "1", "1", "2", "0"], ["484147311015190666  ", "06.05.2015 09:33:00", "1866", "155915", "1", "1", "1", "2", "0"], ["484147311015190158  ", "06.05.2015 09:50:00", "1866", "155915", "1", "1", "1", "12", "0"], ["484147311015180390  ", "06.05.2015 09:50:00", "1866", "155915", "1", "1", "1", "12", "0"], ["484147311015190047  ", "06.05.2015 09:35:00", "1866", "155915", "1", "1", "1", "3", "0"], ["484147311015190460  ", "06.05.2015 09:50:00", "1866", "155915", "1", "1", "1", "12", "0"], ["484147311015190445  ", "06.05.2015 09:45:00", "1866", "155915", "1", "1", "1", "9", "0"], ["484147311015190458  ", "06.05.2015 09:51:00", "1866", "155915", "1", "1", "1", "12", "0"], ["484147311015190448  ", "06.05.2015 09:52:00", "1866", "155915", "1", "1", "1", "13", "0"], ["484147311015190456  ", "06.05.2015 09:53:00", "1866", "155915", "1", "1", "1", "13", "0"], ["484147311015190450  ", "06.05.2015 09:36:00", "1866", "155915", "1", "1", "1", "4", "0"], ["484147311015190461  ", "06.05.2015 09:43:00", "1866", "155915", "1", "1", "1", "8", "0"], ["484147311015190447  ", "06.05.2015 09:52:00", "1866", "155915", "1", "1", "1", "13", "0"], ["484147311015190455  ", "06.05.2015 09:50:00", "1866", "155915", "1", "1", "1", "12", "0"], ["484147311015190454  ", "06.05.2015 09:53:00", "1866", "155915", "1", "1", "1", "13", "0"], ["484147311015190449  ", "06.05.2015 09:43:00", "1866", "155915", "1", "1", "1", "8", "0"], ["484147311015190451  ", "06.05.2015 09:46:00", "1866", "155915", "1", "1", "1", "10", "0"], ["484147311015190457  ", "06.05.2015 09:35:00", "1866", "155915", "1", "1", "1", "3", "0"], ["484147311015190468  ", "06.05.2015 09:43:00", "1866", "155915", "1", "1", "1", "8", "0"], ["484147311015190452  ", "06.05.2015 09:34:00", "1866", "155915", "1", "1", "1", "2", "0"], ["484147311015190481  ", "06.05.2015 09:47:00", "1866", "155915", "1", "1", "1", "10", "0"], ["484147311015190484  ", "06.05.2015 09:37:00", "1866", "155915", "1", "1", "1", "4", "0"], ["484147311015190497  ", "06.05.2015 09:49:00", "1866", "155915", "1", "1", "1", "12", "0"], ["484147311015190498  ", "06.05.2015 09:47:00", "1866", "155915", "1", "1", "1", "10", "0"], ["484147311015190500  ", "06.05.2015 09:38:00", "1866", "155915", "1", "1", "1", "5", "0"], ["484147311015190495  ", "06.05.2015 09:38:00", "1866", "155915", "1", "1", "1", "5", "0"], ["484147311015190470  ", "06.05.2015 09:37:00", "1866", "155915", "1", "1", "1", "4", "0"], ["484147311015190472  ", "06.05.2015 09:47:00", "1866", "155915", "1", "1", "1", "10", "0"], ["484147311015190467  ", "06.05.2015 09:48:00", "1866", "155915", "1", "1", "1", "11", "0"], ["484147311015190493  ", "06.05.2015 09:49:00", "1866", "155915", "1", "1", "1", "11", "0"], ["484147311015190494  ", "06.05.2015 09:48:00", "1866", "155915", "1", "1", "1", "11", "0"], ["484147311015190469  ", "06.05.2015 09:37:00", "1866", "155915", "1", "1", "1", "4", "0"], ["484147311015190492  ", "06.05.2015 09:47:00", "1866", "155915", "1", "1", "1", "10", "0"], ["484147311015190471  ", "06.05.2015 09:38:00", "1866", "155915", "1", "1", "1", "5", "0"], ["484147311015190474  ", "06.05.2015 09:43:00", "1866", "155915", "1", "1", "1", "8", "0"], ["484147311015190491  ", "06.05.2015 09:36:00", "1866", "155915", "1", "1", "1", "3", "0"], ["484147311015190490  ", "06.05.2015 09:38:00", "1866", "155915", "1", "1", "1", "5", "0"], ["484147311015190489  ", "06.05.2015 09:35:00", "1866", "155915", "1", "1", "1", "3", "0"], ["484147311015190488  ", "06.05.2015 09:53:00", "1866", "155915", "1", "1", "1", "13", "0"], ["484147311015190475  ", "06.05.2015 09:49:00", "1866", "155915", "1", "1", "1", "11", "0"], ["484147311015190476  ", "06.05.2015 09:36:00", "1866", "155915", "1", "1", "1", "4", "0"], ["484147311015190487  ", "06.05.2015 09:49:00", "1866", "155915", "1", "1", "1", "11", "0"], ["484147311015190486  ", "06.05.2015 09:54:00", "1866", "155915", "1", "1", "1", "14", "0"], ["484147311015190478  ", "06.05.2015 09:36:00", "1866", "155915", "1", "1", "1", "4", "0"], ["484147311015190480  ", "06.05.2015 09:35:00", "1866", "155915", "1", "1", "1", "3", "0"], ["484147311015190477  ", "06.05.2015 09:35:00", "1866", "155915", "1", "1", "1", "3", "0"], ["484147311015190499  ", "06.05.2015 09:50:00", "1866", "155915", "1", "1", "1", "12", "0"], ["484147311015190485  ", "06.05.2015 09:35:00", "1866", "155915", "1", "1", "1", "3", "0"], ["484147311015190483  ", "06.05.2015 09:36:00", "1866", "155915", "1", "1", "1", "4", "0"], ["484147311015190479  ", "06.05.2015 09:38:00", "1866", "155915", "1", "1", "1", "5", "0"], ["484147311015190453  ", "06.05.2015 09:38:00", "1866", "155915", "1", "1", "1", "5", "0"], ["484147311015190516  ", "06.05.2015 09:49:00", "1866", "155915", "1", "1", "1", "11", "0"], ["484147311015190532  ", "06.05.2015 09:52:00", "1866", "155915", "1", "1", "1", "13", "0"], ["484147311015190530  ", "06.05.2015 09:36:00", "1866", "155915", "1", "1", "1", "3", "0"], ["484147311015190528  ", "06.05.2015 09:50:00", "1866", "155915", "1", "1", "1", "12", "0"], ["484147311015190515  ", "06.05.2015 09:35:00", "1866", "155915", "1", "1", "1", "3", "0"], ["484147311015190514  ", "06.05.2015 09:36:00", "1866", "155915", "1", "1", "1", "4", "0"], ["484147311015190513  ", "06.05.2015 09:49:00", "1866", "155915", "1", "1", "1", "11", "0"], ["484147311015190510  ", "06.05.2015 09:37:00", "1866", "155915", "1", "1", "1", "4", "0"], ["484147311015190523  ", "06.05.2015 09:37:00", "1866", "155915", "1", "1", "1", "4", "0"], ["484147311015190509  ", "06.05.2015 09:40:00", "1866", "155915", "1", "1", "1", "6", "0"], ["484147311015190526  ", "06.05.2015 09:32:00", "1866", "155915", "1", "1", "1", "1", "0"]]) -> (2 "nombreCartons":i32, 3 "triParCarton":string[][](array[string]))   [LabVIEW 2020]
panel:
  out "taille(s) 2":i32[](array[numeric])
  out "taille(s)":i32[](array[numeric])
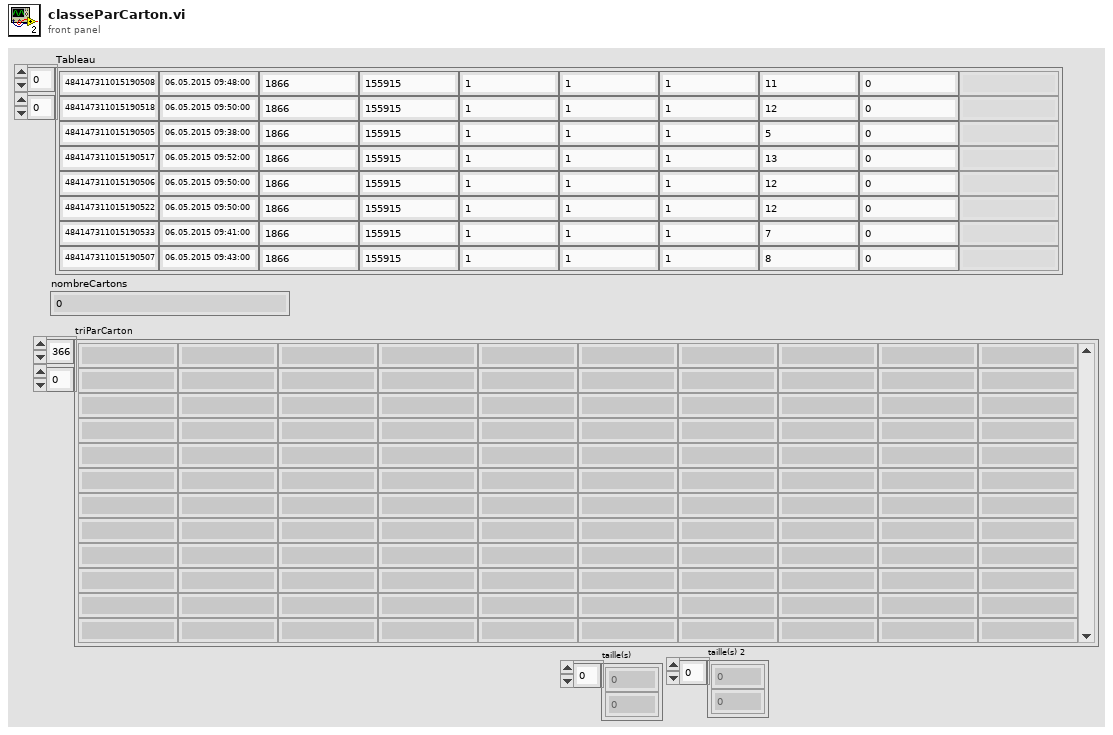
[diagram p1: front panel]
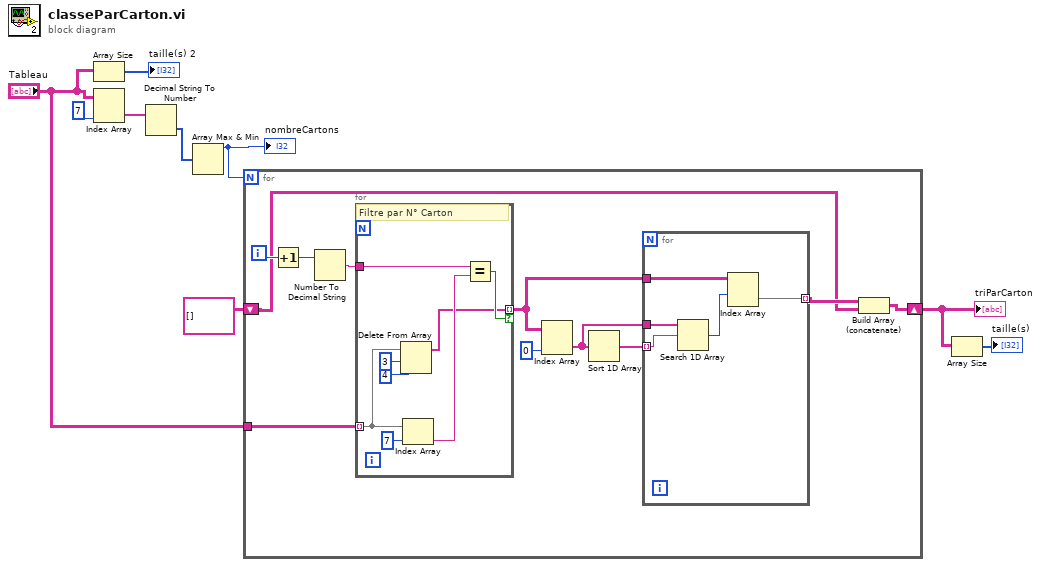
[diagram p0: block diagram]
diagram:
  n1 = Array Size(array="Tableau") -> (size(s)=→"taille(s) 2":i32[])
  n2 = Index Array(array="Tableau", index (col)=7 ("indice")) -> (element=w9:string[])  [unwired: 1 in]
  n3 = Decimal String To Number(string=w9) -> (number=w8:i32[])  [unwired: 2 in, 1 out]
  n4 = Array Max & Min(array=w8) -> (max value=w6:i32)  [unwired: 3 out]
  "nombreCartons" <- w6
  n5 = for {
    N: w6 -> [_]
    tunnel: "Tableau" -> [w20]
    shift-right: [w17] -> w4
    shift-left: string[][] [] -> [w10]
    i -> [w19]
    n6 = Increment(x=w19) -> (x+1=w16:i32)
    n7 = Number To Decimal String(number=w16) -> (decimal integer string=w18:string)  [unwired: 1 in]
    n8 = for {
      tunnel: w20 -> [w29] mode=indexing
      tunnel: w18 -> [w33]
      tunnel: [w26] -> w14 mode=indexing if=w30
      # "Filtre par N° Carton"
      n9 = Delete From Array(array=w29, length=3 ("longueur"), index=4 ("indice")) -> (array with subset deleted=w26:string[])  [unwired: 1 out]
      n10 = Index Array(array=w29, index=7 ("indice")) -> (element=w31:string)
      n11 = Equal?(x=w33, y=w31) -> (x = y?=w30:bool)
    }
    n12 = Index Array(array=w14, index (col)=0 ("indice désactivé (col)")) -> (element=w12:string[])  [unwired: 1 in]
    n13 = Sort 1D Array(array=w12) -> (sorted array=w13:string[])
    n14 = for {
      tunnel: w14 -> [w23]
      tunnel: w13 -> [w24] mode=indexing
      tunnel: w12 -> [w25]
      tunnel: [w21] -> w11 mode=indexing
      n15 = Search 1D Array(1D array=w25, element=w24) -> (index of element=w22:i32)  [unwired: 1 in]
      n16 = Index Array(array=w23, index (row)=w22) -> (element=w21:string[])  [unwired: 1 in]
    }
    n17 = Build Array (concatenate)(w11, w10) -> (w17:string[][])
  }
  "triParCarton" <- w4
  n18 = Array Size(array=w4) -> (size(s)=→"taille(s)":i32[])
